vi "PM103 100kS per second Sample.vi"() -> ()   [LabVIEW 2019]
panel:
  out "Data":cluster{"Empy Time":u32[], "Empty Data":dbl[]}(graph)
  in  "Empty Data":dbl[](array[numeric])
  in  "Empy Time":u32[](array[numeric])
  out "Active":bool
  # "Thorlabs Power Meter Series\n   PM103 100kS/s example"
  # "This example will connect the first found power meter.\nThis will start a measurement with the PM103 for 3 seconds\nat 100kS/s.\nThe time is in microseconds."
  # "Connected"
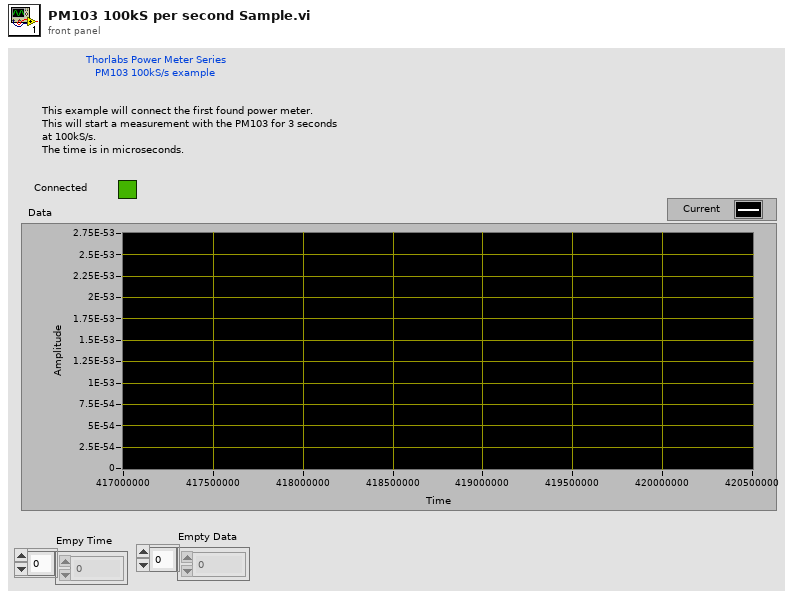
[diagram p1: front panel]
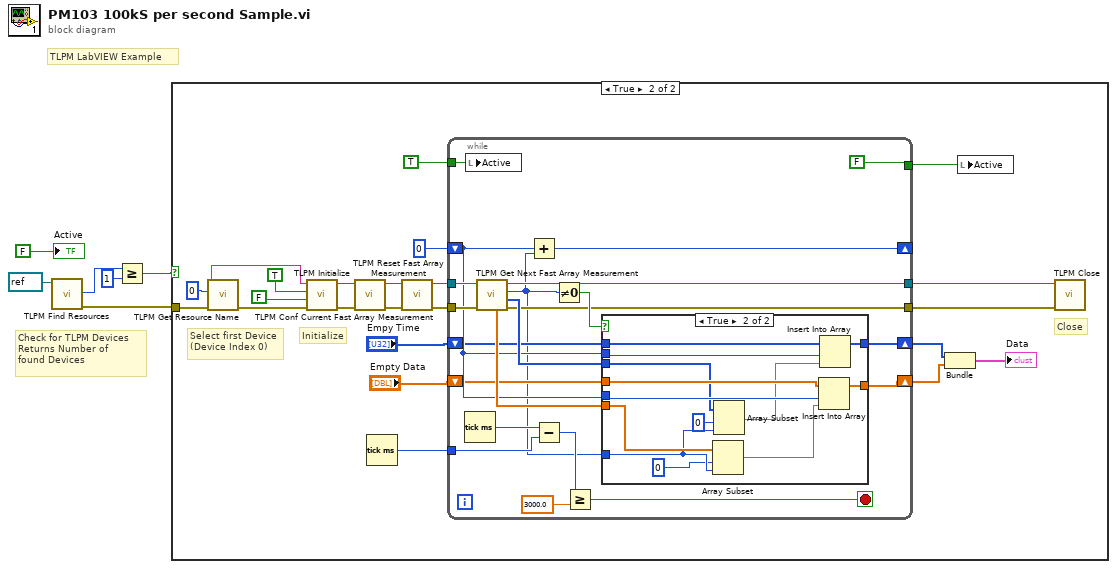
[diagram p0: block diagram]
diagram:
  # "Check for TLPM Devices\nReturns Number of\nfound Devices"
  # "TLPM LabVIEW Example"
  n1 = call <instrlib>:"TLPM Find Resources.vi"("instrument handle"=refnum<visa-resource-name> refnum) -> ("error out"=w3:errorcluster, "Resource Count"=w5:u32)  [unwired: 8 in, 1 out]
  n2 = Greater Or Equal?(x=w5, y=u32 1) -> (x >= y?=w2:bool)
  n3 = case shown="True" w2 {
    tunnel: w3 -> [_ w24]
    frame False {
    }
    frame True {
      # "Close"
      # "Initialize"
      # "Select first Device\n(Device Index 0)"
      n4 = call <instrlib>:"TLPM Get Resource Name.vi"("error in (no error)"=w24, "Index (0)"=u32 0 ("Device Index")) -> ("error out"=w29:errorcluster, "Resource Name"=w28:string)  [unwired: 7 in, 1 out]
      n5 = call <instrlib>:"TLPM Initialize.vi"("error in (no error)"=w29, "Reset Device (Reset Device)"=FALSE ("ID Query (Do Query)"), "ID Query (Do Query)"=TRUE, "resource name"=w28) -> ("error out"=w10:errorcluster, "instrument handle out"=w9:refnum<visa-resource-name>)  [unwired: 6 in]
      n6 = call <instrlib>:"TLPM Reset Fast Array Measurement.vi"("error in (no error)"=w10, "instrument handle"=w9) -> ("error out"=w7:errorcluster, "instrument handle out"=w8:refnum<visa-resource-name>)  [unwired: 8 in]
      n7 = Tick Count (ms)() -> (millisecond timer value=w17:u32)
      n8 = call <instrlib>:"TLPM Conf Current Fast Array Measurement.vi"("error in (no error)"=w7, "instrument handle"=w8) -> ("error out"=w20:errorcluster, "instrument handle out"=w21:refnum<visa-resource-name>)  [unwired: 8 in]
      n9 = while {
        tunnel: TRUE -> [w50]
        tunnel: [FALSE] -> w22
        tunnel: w21 -> [w47]
        tunnel: w20 -> [w48]
        tunnel: [w31] -> w19
        tunnel: [w38] -> w18
        tunnel: w17 -> [w46]
        shift-right: [w37] -> _
        shift-left: u16 0 ("Count") -> [w36]
        shift-right: [w35] -> w13
        shift-left: "Empy Time" -> [w34]
        shift-right: [w33] -> w12
        shift-left: "Empty Data" -> [w32]
        stop <- w42 stop-if-true
        n10 = Tick Count (ms)() -> (millisecond timer value=w45:u32)
        n11 = local write "Active"(w50) -> ()
        n12 = call <instrlib>:"TLPM Get Next Fast Array Measurement.vi"("error in (no error)"=w48, "instrument handle"=w47) -> ("error out"=w38:errorcluster, "Timestamps"=w39:u32[], "Count"=w30:u16, "instrument handle out"=w31:refnum<visa-resource-name>, "Meas Data"=w40:dbl[])  [unwired: 5 in]
        n13 = Add(x=w36, y=w30) -> (x+y=w37:u16)
        n14 = Subtract(x=w45, y=w46) -> (x-y=w43:u32)
        n15 = Not Equal To 0?(x=w30) -> (x != 0?=w41:bool)
        n16 = Greater Or Equal?(x=w43, y=3000.0) -> (x >= y?=w42:bool)
        n17 = case shown="True" w41 {
          tunnel: w40 -> [_ w59]
          tunnel: w39 -> [_ w58]
          tunnel: w36 -> [_ w65]
          tunnel: w36 -> [_ w64]
          tunnel: [w52 w63] -> w35
          tunnel: w34 -> [w52 w62]
          tunnel: [w51 w61] -> w33
          tunnel: w32 -> [w51 w60]
          tunnel: w30 -> [_ w57]
          frame False {
          }
          frame True {
            n18 = Array Subset(array=w59, index=0, length=w57) -> (w53:dbl[])
            n19 = Array Subset(array=w58, index=0, length=w57) -> (w54:u32[])
            n20 = Insert Into Array(array=w60, index=w64, new element=w53) -> (w61:dbl[])
            n21 = Insert Into Array(array=w62, index=w65, new element=w54) -> (w63:u32[])
          }
        }
      }
      n22 = Bundle("Empy Time"=w13, "Empty Data"=w12) -> (→"Data":cluster{"Empy Time":u32[], "Empty Data":dbl[]})  [unwired: 1 in]
      n23 = local write "Active"(w22) -> ()
      n24 = call <instrlib>:"TLPM Close.vi"("error in (no error)"=w18, "instrument handle"=w19) -> ()  [unwired: 9 in, 1 out]
    }
  }
  "Active" <- FALSE ("Active")
